vi "scan time(SubVI).vi"(0 "total time":dbl=10.0, 9 "steps number":i32, 12 "data":refnum<queue>, 14 "config":refnum<queue>) -> (6 "错误输出":errorcluster)   [LabVIEW 2019, in "SubVI.lvlib"]
uses:
  SubVI.lvlib
  config.ctl
  Instrument.ctl
  lib/QDInstrument.dll
  <vilib>/NI/Modbus Library/API/Master/Modbus Master.lvclass
panel:
  # "(真是通道1，假是通道2)"
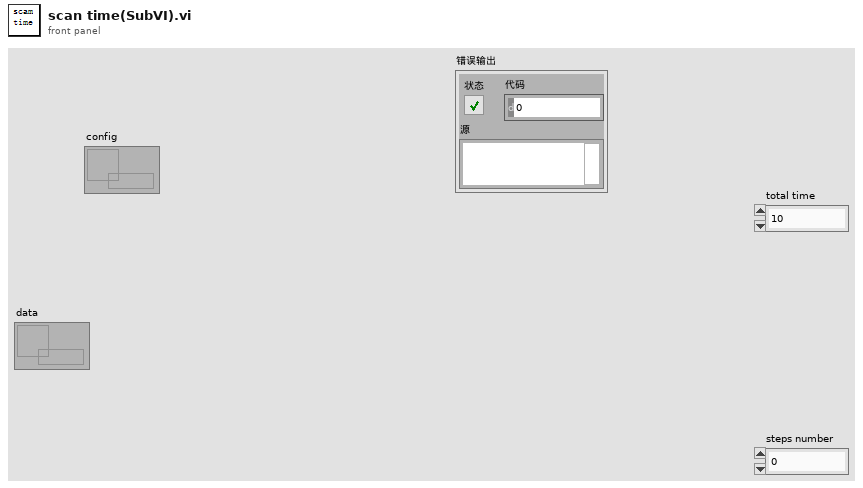
[diagram p1: front panel]
types:
  T1 = typedef "config.ctl" = cluster{"initialize":string, "6221":cluster{"6221 Resource":refnum<visa-resource-name>, "Delta status":bool}, "7001":cluster{"Ch":bool}, "SR830+6221":cluster{"source":u16, "阻抗":dbl, "量程入 4":i32, "量程入 3":i32, "量程入 2":i32, "量程入 1":i32, "电流":dbl, "SR830 2":bool, "SR830 3":bool, "SR830 4":bool, "SR830 1":bool, "VISA 1":refnum<visa-resource-name>, "VISA 2":refnum<visa-resource-name>, "VISA 3":refnum<visa-resource-name>, "VISA 4":refnum<visa-resource-name>, "量程":enum16{"量程每次测量会判定", "量程不变为设定值"}}, "2400":cluster{"2400":bool, "VISA":refnum<visa-resource-name>}, "ch":cluster{"ch str":string, "ch1":bool, "ch2":bool, "布尔":bool}, "error":bool, "数据文件路径":path, "log":cluster{"log路径":path, "log interval":dbl}, "Instrument":T2}
  T2 = typedef "Instrument.ctl" = cluster{"335 Resource":refnum<visa-resource-name>, "Input (0:A)":u16, "Instrument Type":i32, "quantum design":refnum<k24>, "Heater Output (1:1)":u16, "335state":refnum<vi>, "semaphore":T3, "TCP master instance":refnum<class "Modbus Master.lvclass">}
  T3 = typedef "Semaphore RefNum" = refnum<k1>
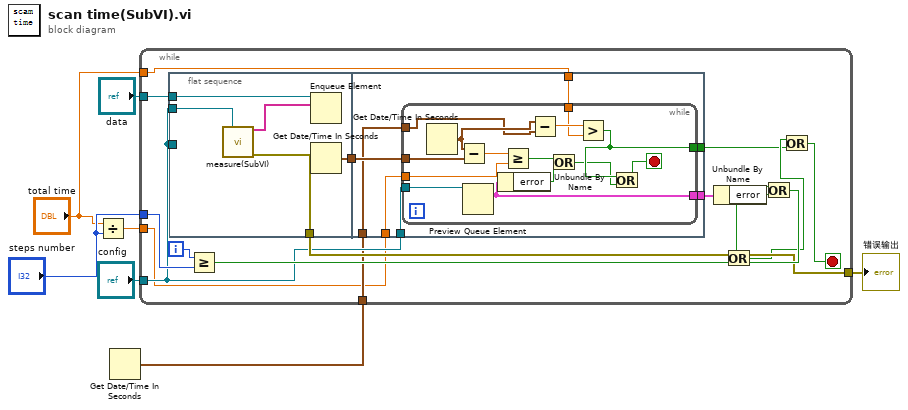
[diagram p0: block diagram]
diagram:
  n1 = Divide(x="total time", y="steps number") -> (x/y=w6:dbl)
  n2 = Get Date/Time In Seconds() -> (seconds since 1Jan1904=w2:timestamp)
  n3 = while {
    tunnel: "steps number" -> [w21]
    tunnel: "data" -> [w23]
    tunnel: w6 -> [w12]
    tunnel: [w17] -> w5
    tunnel: "config" -> [w16]
    tunnel: w2 -> [w13]
    tunnel: "total time" -> [w8]
    i -> [w20]
    stop <- w9 stop-if-true
    n4 = flat-sequence {
      tunnel: w23 -> [w28]
      tunnel: w16 -> [w27]
      tunnel: w16 -> [_]
      tunnel: [w26] -> w17
      tunnel: [w24] -> w18
      tunnel: w16 -> [w33]
      tunnel: [w32] -> w15
      tunnel: w12 -> [w34]
      tunnel: w18 -> [w35]
      tunnel: w13 -> [w31]
      tunnel: w8 -> [w30]
      tunnel: [w29] -> w10
      frame #0 {
        n5 = call "measure(SubVI).vi"("config"=w27) -> ("data"=w25:string[], "error out"=w26:errorcluster)  [unwired: 13 in]
        n6 = Enqueue Element(queue=w28, element=w25) -> ()  [unwired: 2 in, 3 out]
        n7 = Get Date/Time In Seconds() -> (seconds since 1Jan1904=w24:timestamp)
      }
      frame #1 {
        n8 = while {
          tunnel: w35 -> [w45]
          tunnel: w34 -> [w48]
          tunnel: w33 -> [w47]
          tunnel: [w44] -> w32
          tunnel: w31 -> [w41]
          tunnel: w30 -> [w39]
          tunnel: [w38] -> w29
          stop <- w36 stop-if-true
          n9 = Get Date/Time In Seconds() -> (seconds since 1Jan1904=w42:timestamp)
          n10 = Subtract(x=w42, y=w45) -> (x-y=w49:dbl)
          n11 = Preview Queue Element(queue=w47) -> (element=w44:T1)  [unwired: 2 in, 3 out]
          n12 = Unbundle By Name(w44) -> ("error"=w43:bool)
          n13 = Greater Or Equal?(x=w49, y=w48) -> (x >= y?=w46:bool)
          n14 = Subtract(x=w42, y=w41) -> (x-y=w40:dbl)
          n15 = Or(x=w46, y=w43) -> (x .or. y?=w37:bool)
          n16 = Greater?(x=w40, y=w39) -> (0:w38:bool)
          n17 = Or(x=w38, y=w37) -> (x .or. y?=w36:bool)
        }
      }
    }
    n18 = Greater Or Equal?(x=w20, y=w21) -> (x >= y?=w22:bool)
    n19 = Unbundle By Name(w15) -> ("error"=w14:bool)
    n20 = Or(x=w22, y=w14) -> (x .or. y?=w19:bool)
    n21 = Or(x=w17, y=w19) -> (x .or. y?=w11:bool)
    n22 = Or(x=w11, y=w10) -> (x .or. y?=w9:bool)
  }
  "错误输出" <- w5
